vi "MoveAbs.vi"(8 "error in":errorcluster, 9 "Axis":i32, 10 "Position":dbl, 11 "VISA resource":refnum<visa-resource-name>) -> (0 "error out":errorcluster)   [LabVIEW 2012, in "Micos_uic.lvlib"]
uses:
  Micos_uic.lvlib
  Position_Micos.vi
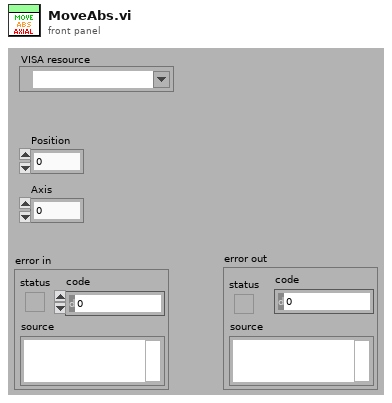
[diagram p1: front panel]
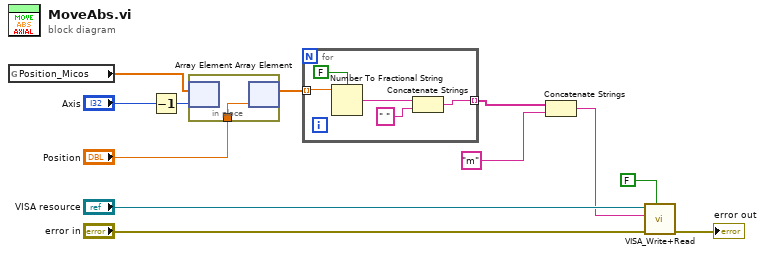
[diagram p0: block diagram]
diagram:
  n1 = global read "Position_Micos.vi" "Position_Micos"() -> (w2:dbl[])
  n2 = Decrement(x="Axis") -> (x-1=w8:i32)
  n3 = in-place {
    in-place-border: "Position" -> [w13]
    n4 = in-place-array #1(w2, w8) -> ()  [unwired: 1 out]
    n5 = in-place-array #1(w13) -> (w6:dbl[])  [unwired: 1 out]
  }
  n6 = for {
    tunnel: w6 -> [w18] mode=indexing
    tunnel: [w14] -> w3 mode=indexing
    n7 = Number To Fractional String(use system decimal point (T)=FALSE, number=w18) -> (F-format string=w16:string)  [unwired: 2 in]
    n8 = Concatenate Strings(w16, " " ("string")) -> (w14:string)
  }
  n9 = Concatenate Strings(w3, "m" ("format string")) -> (w4:string)
  n10 = call "VISA_Write+Read.vi"("Read?"=FALSE, "error in (no error)"="error in", "Write Buffer"=w4, "VISA resource name"="VISA resource") -> ("error out"=→"error out":errorcluster)  [unwired: 5 in, 2 out]
